vi "Place Front Gear.vi"(8 "error in":errorcluster) -> (0 "error out":errorcluster)   [LabVIEW 2016]
uses:
  Refname/Motors.ctl
  Refname/Refname to String (Motors).vi
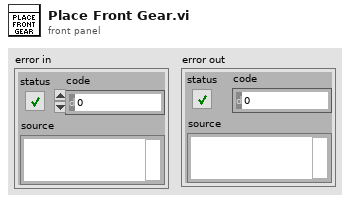
[diagram p1: front panel]
types:
  T1 = typedef "Motors.ctl" = enum16{"Wheel 1", "Swerve 1", "Wheel 2", "Swerve 2", "Wheel 3", "Swerve 3", "Wheel 4", "Swerve 4", "Climber"}
  T2 = typedef "WPI_MotorControlDeviceRef.ctl" = cluster{"DeviceStatus":errorcluster, "Type":T3, "PWM":cluster{"PWM Channel":T4, "DeadBand":T5}, "CAN":cluster{"Device Number":u8, "SetOutput VI Ref":variant, "GetOutput VI Ref":variant, "Enable VI Ref":variant, "Disable VI Ref":variant, "Data":variant}, "Invert":bool}
  T3 = typedef "WPI_MotorControlType.ctl" = enum16{"PWM", "CAN"}
  T4 = typedef "FPGA_DIOPWMChannel.ctl" = enum8{"PWM 0", "PWM 1", "PWM 2", "PWM 3", "PWM 4", "PWM 5", "PWM 6", "PWM 7", "PWM 8", "PWM 9", "PWM MXP 0", "PWM MXP 1", "PWM MXP 2", "PWM MXP 3", "PWM MXP 4", "PWM MXP 5", "PWM MXP 6", "PWM MXP 7", "PWM MXP 8", "PWM MXP 9", "Invalid"}
  T5 = typedef "WPI_PWMDeadband.ctl" = cluster{"Name":string, "maxPositivePwm":i32, "minPositivePwm":i32, "centerPwm":i32, "maxNegativePwm":i32, "minNegativePwm":i32, "angularRange":u16}
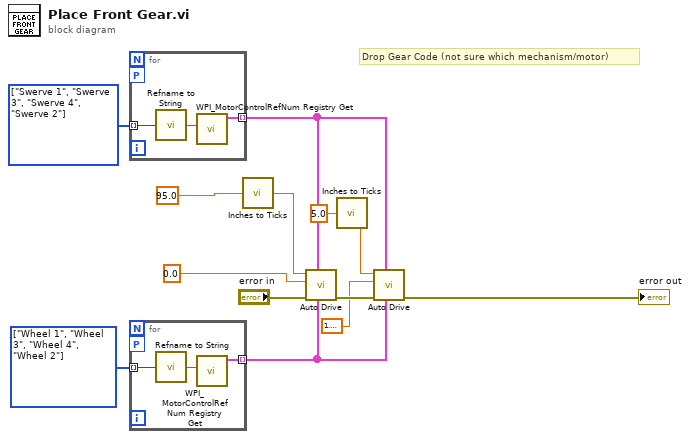
[diagram p0: block diagram]
diagram:
  w11 = T1[] [enum."Wheel 1", enum."Wheel 3", enum."Wheel 4", enum."Wheel 2"] items=["Wheel 1", "Swerve 1", "Wheel 2", "Swerve 2", "Wheel 3", "Swerve 3", "Wheel 4", "Swerve 4", "Climber"]
  w12 = T1[] [enum."Swerve 1", enum."Swerve 3", enum."Swerve 4", enum."Swerve 2"] items=["Wheel 1", "Swerve 1", "Wheel 2", "Swerve 2", "Wheel 3", "Swerve 3", "Wheel 4", "Swerve 4", "Climber"]
  # "Drop Gear Code (not sure which mechanism/motor)"
  n1 = for {
    workers-P: _ -> [_]
    tunnel: w12 -> [w16] mode=indexing
    tunnel: [w14] -> w6 mode=indexing
    n2 = call-poly "Refname to String.vi"("Enum"=w16) -> ("String"=w15:string)
    n3 = call <vilib>:"WPI_MotorControlRefNum Registry Get.vi"("refnum name"=w15) -> ("MotorControlDevRef"=w14:T2)  [unwired: 9 in, 1 out]
  }
  n4 = for {
    workers-P: _ -> [_]
    tunnel: w11 -> [w19] mode=indexing
    tunnel: [w17] -> w7 mode=indexing
    n5 = call-poly "Refname to String.vi"("Enum"=w19) -> ("String"=w18:string)
    n6 = call <vilib>:"WPI_MotorControlRefNum Registry Get.vi"("refnum name"=w18) -> ("MotorControlDevRef"=w17:T2)  [unwired: 9 in, 1 out]
  }
  n7 = call "Inches to Ticks.vi"("Inches"=95.0 ("Distance(in)")) -> ("Ticks"=w9:dbl)
  n8 = call "Auto Drive.vi"("Wheel DevRef"=w7, "Swerve DevRef"=w6, "error in"="error in", "Drive Angle"=0.0 ("Drive Angle (radian)"), "Ticks(Distance)"=w9) -> ("error out"=w8:errorcluster)  [unwired: 6 in]
  n9 = call "Inches to Ticks.vi"("Inches"=5.0) -> ("Ticks"=w3:dbl)
  n10 = call "Auto Drive.vi"("Wheel DevRef"=w7, "Swerve DevRef"=w6, "error in"=w8, "Drive Angle"=1.5707963267948966, "Ticks(Distance)"=w3) -> ("error out"=→"error out":errorcluster)  [unwired: 6 in]
